vi "Main_progetto.vi"() -> ()   [LabVIEW 2019]
uses:
  <vilib>/Analysis/coordinate.llb/Angle Units.ctl
  <vilib>/Analysis/coordinate.llb/Angle Range (Degree).ctl
  <vilib>/Analysis/coordinate.llb/Wrap Angle (scalar).vi
  <vilib>/Analysis/coordinate.llb/Wrap Angle (array).vi
  <vilib>/Analysis/4window.llb/Triangle Window (DBL).vi
  <vilib>/Analysis/4window.llb/Hanning Window (DBL).vi
  <vilib>/Analysis/2dsp.llb/Real FFT.vi
  <vilib>/Analysis/4window.llb/AllCosWindow (DBL).vi
  <vilib>/Utility/file.llb/Write Delimited Spreadsheet (string).vi
  <vilib>/measure/NI_MABase.lvlib
  <vilib>/Analysis/NI_AALBase.lvlib
  <vilib>/Analysis/NI_AAL_Angle.lvlib
  <vilib>/Analysis/NI_AALPro.lvlib
panel:
  in  "IpDFT?":bool
  in  "Tw [s]":dbl=0.04
  in  "Finestra":enum16{"Rettangolare", "Triangolare", "Hann"}(ring)=enum."Hann"
  in  "Tab Control":T1(tab)=enum."Finestratura e DFT"
  in  "Gradino_FASE?":bool
  in  "Gradi innalzamento[°]":dbl=10.0
  in  "Gradino_AMP?":bool
  in  "Variazione Percentuale [%]":dbl=10.0
  in  "t0[s]":dbl=1.0
  in  "f_mp":dbl=5.0
  in  "f_ma":dbl=5.0
  in  "Ka":dbl
  in  "Kx":dbl=0.1
  out "Segnale + Fronti PPS":waveform(dbl)[](graph)=[{"t0"=timestamp(3664183274 s since 1904-01-01), "dt"=0.0001, "Y"=array[10000 elements]}, {"t0"=timestamp(3664183274 s since 1904-01-01), "dt"=0.0001, "Y"=array[10000 elements]}]
  in  "Tipo di Segnale":T2(ring)
  in  "#PPS":dbl=50.0
  in  "Tempo Osservazione [s]":dbl=1.0
  in  "fs [Campioni/s]":i32=10000
  in  "Fase iniziale [°]":dbl
  in  "Frequenza [Hz]":dbl=50.0
  in  "Ampiezza [V]":dbl=5.0
  out "#Campioni":dbl=10000.0
  out "Indici Fronte PPS":i32[](array[numeric])=[200, 400, 600, 800, 1000, 1200, 1400, 1600, 1800, 2000, 2200, 2400, 2600, 2800, 3000, 3200, 3400, 3600, 3800, 4000, 4200, 4400, 4600, 4800, 5000, 5200, 5400, 5600, 5800, 6000, 6200, 6400, 6600, 6800, 7000, 7200, 7400, 7600, 7800, 8000, 8200, 8400, 8600, 8800, 9000, 9200, 9400, 9600, 9800]
  out "Ampiezza":waveform(dbl)(graph)={"t0"=timestamp(3664183274 s since 1904-01-01), "dt"=0.0001, "Y"=array[10000 elements]}
  out "Fase":waveform(dbl)(graph)={"t0"=timestamp(3664183274 s since 1904-01-01), "dt"=0.0001, "Y"=array[10000 elements]}
  out "Frequenza":waveform(dbl)(graph)={"t0"=timestamp(3664183274 s since 1904-01-01), "dt"=0.0001, "Y"=array[10000 elements]}
  out "current time":timestamp=timestamp(3664183274 s since 1904-01-01)
  in  "Ampiezza [% Fondamentale]":dbl=10.0
  in  "Indice Fondamentale":i32=2
  in  "Armonica?":bool
  in  "Fase Arm [°]":dbl=90.0
  in  "Rumore?":bool
  in  "SNR[dB]":dbl=20.0
  out "tf":dbl
  in  "Rf":dbl=1.0
  in  "f1":dbl=45.0
  in  "f2":dbl=55.0
  in  "ti":dbl=1.0
  out "#cicli nominali in Tw":dbl=2.0
  out "FFT Modulo":dbl[](graph)=[0.2004284654332121, 0.2771875769031888, 2.4289122109023182, 0.14855120479340944, 0.06711997171608222, 0.040910071789265014, 0.02860978087861402, 0.021693180356150216, 0.01735076197275401, 0.014410410758733146, 0.012305673610300686, 0.010733350016924947, 0.00951833235799889, 0.00855331737321674, 0.007769333424100193, 0.007120260807923017, 0.0065742159898430855, 0.006108519981725259, 0.005706637938963746, 0.00535625155471345, 0.005048007477321536, 0.004774682642835479, 0.004530614276304571, 0.004311302288502253, 0.004113126580084852, 0.00393314254154195, 0.003768930776703592, 0.003618485076706068, 0.0034801278028881856, 0.003352445195024498, 0.0032342373581623067, 0.0031244791961971886, 0.0030222896028904455, 0.0029269069476381758, 0.002837669407508284, 0.0027539990648302085, 0.002675388955918328, 0.002601392451414109, 0.0025316144927998267, 0.0024657043171863423, 0.002403349383395278, 0.002344270273936035, 0.002288216394479222, 0.0022349623286919426, 0.0021843047348013493, 0.0021360596917879443, 0.002090060421054105, 0.00204615532277344, 0.0020042062772505946, 0.001964087170384628, 0.0019256826093842281, 0.0018888868006225951, 0.0018536025661511036, 0.0018197404793038816, 0.0017872181027114862, 0.001755959314936195, 0.0017258937138572004, 0.001696956086625786, 0.0016690859379216423, 0.0016422270688726094, 0.001616327200532036, 0.001591337636447327, 0.0015672129596478706, 0.0015439107600185866, 0.0015213913885452437, 0.0014996177353782815, 0.0014785550290975637, 0.0014581706547211013, 0.0014384339886332367, 0.0014193162484461821, 0.0014007903562823843, 0.0013828308142269058, 0.0013654135904523955, 0.0013485160151872353, 0.001332116685420944, 0.0013161953775471433, 0.0013007329671651806, 0.0012857113553683764, 0.001271113400898479, 0.0012569228576905357, 0.0012431243171547128, 0.0012297031550276365, 0.001216645482162153, 0.0012039380989247045, 0.0011915684531612913, 0.0011795246009920425, 0.001167795170576942, 0.001156369328410249, 0.0011452367479786612, 0.0011343875806037183, 0.001123812428279146, 0.001113502318356494, 0.0011034486799218212, 0.0010936433217333095, 0.0010840784116325608, 0.0010747464572455527, 0.001065640287970658, 0.001056753038069751, 0.0010480781308387342, 0.0010396092637684215, 0.0010313403946015805, 0.0010232657282498885, 0.0010153797044930933, 0.001007676986416554, 0.001000152449526727, 0.0009928011715113465, 0.0009856184225786999, 0.0009785996563626902, 0.000971740501352381, 0.000965036752774153, 0.0009584843649591924, 0.0009520794441221284, 0.0009458182415198593, 0.0009396971470064985, 0.0009337126829168997, 0.0009278614982866133, 0.0009221403633728558, 0.0009165461644668986, 0.0009110758989654318, 0.0009057266707131591, 0.0009004956855705209, 0.0008953802472070446, 0.0008903777531326384, 0.0008854856908649937, 0.0008807016343617123, 0.0008760232405762775, 0.0008714482462017238, 0.0008669744645753551, 0.0008625997827203524, 0.0008583221585377279, 0.0008541396181274819, 0.0008500502532454137, 0.0008460522188465611, 0.0008421437308167747, 0.0008383230637082276, 0.0008345885486464955, 0.0008309385713546284, 0.0008273715701607699, 0.0008238860342263808, 0.0008204805017666113, 0.0008171535583750218, 0.0008139038354303445, 0.0008107300085636059, 0.0008076307962000254, 0.0008046049581566672, 0.0008016512943030512, 0.0007987686433104722, 0.0007959558813671575, 0.0007932119210777466, 0.0007905357103051015, 0.0007879262310841407, 0.0007853824986460356, 0.0007829035603848542, 0.0007804884949445779, 0.000778136411309154, 0.0007758464479433901, 0.0007736177719647078, 0.0007714495783565443, 0.0007693410891995958, 0.0007672915529728252, 0.0007653002438213416, 0.0007633664609190352, 0.0007614895278423043, 0.0007596687919177555, 0.0007579036236858507, 0.0007561934163169723, 0.0007545375850835884, 0.0007529355668558493, 0.0007513868196077115, 0.0007498908219539457, 0.0007484470727029584, 0.0007470550904400135, 0.0007457144131051204, 0.0007444245976283224, 0.0007431852195461328, 0.0007419958726416369, 0.0007408561686510532, 0.0007397657368926213, 0.0007387242240051496, 0.0007377312936482901, 0.0007367866262287676, 0.0007358899186506904, 0.0007350408840707933, 0.0007342392516738983, 0.0007334847664536476, 0.0007327771890147256, 0.0007321162953945121, 0.0007315018768564688, 0.0007309337397749528, 0.0007304117054513229, 0.0007299356099701171, 0.0007295053041087158, 0.000729120653183006, 0.0007287815369684133, 0.0007284878495977631, 0.000728239499483278, 0.0007280364092437072, 0.0007278785156508138, 0.0007277657695728192, 0.0007276981359433338, 0.0007276755937394297, 0.0007276981359433338, 0.0007277657695728192, 0.0007278785156508138, 0.0007280364092437072, 0.000728239499483278, 0.0007284878495977631, 0.0007287815369684133, 0.000729120653183006, 0.0007295053041087158, 0.0007299356099701171, 0.0007304117054513229, 0.0007309337397749528, 0.0007315018768564688, 0.0007321162953945121, 0.0007327771890147256, 0.0007334847664536476, 0.0007342392516738983, 0.0007350408840707933, 0.0007358899186506904, 0.0007367866262287676, 0.0007377312936482901, 0.0007387242240051496, 0.0007397657368926213, 0.0007408561686510532, 0.0007419958726416369, 0.0007431852195461328, 0.0007444245976283224, 0.0007457144131051204, 0.0007470550904400135, 0.0007484470727029584, 0.0007498908219539457, 0.0007513868196077115, 0.0007529355668558493, 0.0007545375850835884, 0.0007561934163169723, 0.0007579036236858507, 0.0007596687919177555, 0.0007614895278423043, 0.0007633664609190352, 0.0007653002438213416, 0.0007672915529728252, 0.0007693410891995958, 0.0007714495783565443, 0.0007736177719647078, 0.0007758464479433901, 0.000778136411309154, 0.0007804884949445779, 0.0007829035603848542, 0.0007853824986460356, 0.0007879262310841407, 0.0007905357103051015, 0.0007932119210777466, 0.0007959558813671575, 0.0007987686433104722, 0.0008016512943030512, 0.0008046049581566672, 0.0008076307962000254, 0.0008107300085636059, 0.0008139038354303445, 0.0008171535583750218, 0.0008204805017666113, 0.0008238860342263808, 0.0008273715701607699, 0.0008309385713546284, 0.0008345885486464955, 0.0008383230637082276, 0.0008421437308167747, 0.0008460522188465611, 0.0008500502532454137, 0.0008541396181274819, 0.0008583221585377279, 0.0008625997827203524, 0.0008669744645753551, 0.0008714482462017238, 0.0008760232405762775, 0.0008807016343617123, 0.0008854856908649937, 0.0008903777531326384, 0.0008953802472070446, 0.0009004956855705209, 0.0009057266707131591, 0.0009110758989654318, 0.0009165461644668986, 0.0009221403633728558, 0.0009278614982866133, 0.0009337126829168997, 0.0009396971470064985, 0.0009458182415198593, 0.0009520794441221284, 0.0009584843649591924, 0.000965036752774153, 0.000971740501352381, 0.0009785996563626902, 0.0009856184225786999, 0.0009928011715113465, 0.001000152449526727, 0.001007676986416554, 0.0010153797044930933, 0.0010232657282498885, 0.0010313403946015805, 0.0010396092637684215, 0.0010480781308387342, 0.001056753038069751, 0.001065640287970658, 0.0010747464572455527, 0.0010840784116325608, 0.0010936433217333095, 0.0011034486799218212, 0.001113502318356494, 0.001123812428279146, 0.0011343875806037183, 0.0011452367479786612, 0.001156369328410249, 0.001167795170576942, 0.0011795246009920425, 0.0011915684531612913, 0.0012039380989247045, 0.001216645482162153, 0.0012297031550276365, 0.0012431243171547128, 0.0012569228576905357, 0.001271113400898479, 0.0012857113553683764, 0.0013007329671651806, 0.0013161953775471433, 0.001332116685420944, 0.0013485160151872353, 0.0013654135904523955, 0.0013828308142269058, 0.0014007903562823843, 0.0014193162484461821, 0.0014384339886332367, 0.0014581706547211013, 0.0014785550290975637, 0.0014996177353782815, 0.0015213913885452437, 0.0015439107600185866, 0.0015672129596478706, 0.001591337636447327, 0.001616327200532036, 0.0016422270688726094, 0.0016690859379216423, 0.001696956086625786, 0.0017258937138572004, 0.001755959314936195, 0.0017872181027114862, 0.0018197404793038816, 0.0018536025661511036, 0.0018888868006225951, 0.0019256826093842281, 0.001964087170384628, 0.0020042062772505946, 0.00204615532277344, 0.002090060421054105, 0.0021360596917879443, 0.0021843047348013493, 0.0022349623286919426, 0.002288216394479222, 0.002344270273936035, 0.002403349383395278, 0.0024657043171863423, 0.0025316144927998267, 0.002601392451414109, 0.002675388955918328, 0.0027539990648302085, 0.002837669407508284, 0.0029269069476381758, 0.0030222896028904455, 0.0031244791961971886, 0.0032342373581623067, 0.003352445195024498, 0.0034801278028881856, 0.003618485076706068, 0.003768930776703592, 0.00393314254154195, 0.004113126580084852, 0.004311302288502253, 0.004530614276304571, 0.004774682642835479, 0.005048007477321536, 0.00535625155471345, 0.005706637938963746, 0.006108519981725259, 0.0065742159898430855, 0.007120260807923017, 0.007769333424100193, 0.00855331737321674, 0.00951833235799889, 0.010733350016924947, 0.012305673610300686, 0.014410410758733146, 0.01735076197275401, 0.021693180356150216, 0.02860978087861402, 0.040910071789265014, 0.06711997171608222, 0.14855120479340944, 2.4289122109023182, 0.2771875769031888]
  in  "Freq Nom [Hz]":dbl=50.0
  out "Finestre":dbl[][](graph)
  out "Nw":i32=400
  out "Errore Ampiezza":waveform(dbl)(graph)={"t0"=timestamp(3664183274 s since 1904-01-01), "dt"=0.02, "Y"=[-2.783764844462926, -2.0643275081794954, -1.0948068040687353, -0.1185268667778594, 0.6260382249297258, 0.9612665795103048, 0.8083537049149925, 0.2031572038769447, -0.7109376274646095, -1.7128090786989603, -2.553584527277426, -3.018941014895642, -2.9880383189683712, -2.468950838768471, -1.5962499435632438, -0.5917665408033912, 0.2957958814533157, 0.8523582805366736, 0.9463029139744528, 0.5556087136146104, -0.22777463298394807, -1.2165051574097774, -2.1682944281056216, -2.8435115639072883, -3.0682120621809794, -2.783764844462926, -2.0643275081794776, -1.0948068040687708, -0.11852686677787716, 0.6260382249297258, 0.9612665795103226, 0.8083537049149925, 0.2031572038769447, -0.7109376274645918, -1.7128090786989425, -2.553584527277444, -3.018941014895624, -2.9880383189683712, -2.468950838768471, -1.5962499435632616, -0.591766540803409, 0.2957958814533157, 0.8523582805366381, 0.9463029139744883, 0.5556087136146282, -0.22777463298389478, -1.2165051574097419, -2.1682944281056926, -2.8435115639072706]}
  out "Errore Fase":waveform(dbl)(graph)={"t0"=timestamp(3664183274 s since 1904-01-01), "dt"=0.02, "Y"=[-0.9924999827672032, -1.7110408606274774, -1.9782950781677577, -1.7401357120577998, -1.0674646300828705, -0.12793342028531995, 0.8562237454428079, 1.6540002345176053, 2.0717014022732627, 1.9972557434297045, 1.4354923368755657, 0.5196901501313356, -0.5154977010656481, -1.3996886023500466, -1.907559062866504, -1.9206641317435214, -1.4494430035050243, -0.6179136942558117, 0.37334049987567397, 1.291927161654316, 1.9197643004517762, 2.098729550599465, 1.771865154751795, 1.0089419265595867, 1.0132179603049215e-13, -0.9924999827664926, -1.711040860628188, -1.9782950781673136, -1.7401357120615302, -1.0674646300826929, -0.12793342028372123, 0.8562237454401211, 1.6540002345162952, 2.071701402273396, 1.997255743427706, 1.4354923368743222, 0.5196901501328899, -0.5154977010668915, -1.399688602349869, -1.9075590628678363, -1.9206641317449424, -1.4494430035063566, -0.6179136942584762, 0.3733404998801815, 1.2919271616545158, 1.919764300447624, 2.0987295505939474, 1.7718651547519726, 1.00894192655972]}
  out "TVE (Total vector error)":waveform(dbl)(graph)={"t0"=timestamp(3664183274 s since 1904-01-01), "dt"=0.02, "Y"=[2.9507581085918675, 2.6699442744155264, 2.2515062053425523, 1.7431166101168498, 1.2403738519873968, 0.9698235534221632, 1.180032412638305, 1.6680782166788377, 2.183280452227935, 2.618070021606387, 2.9204070891337692, 3.0620138182269923, 3.0308695047565517, 2.8295662779157382, 2.475601509722746, 2.0042942995676443, 1.481403950898688, 1.054317408745175, 1.0179347508680092, 1.4096194593664053, 1.9310278865612676, 2.4147065727130195, 2.7879836372364273, 3.0124022833472104, 3.0682120621809794, 2.9507581085916126, 2.669944274415972, 2.2515062053421486, 1.7431166101206395, 1.2403738519872842, 0.9698235534219634, 1.180032412636331, 1.6680782166775265, 2.1832804522280598, 2.6180700216048662, 2.9204070891332026, 3.062013818227213, 3.0308695047567613, 2.829566277915625, 2.4756015097237265, 2.0042942995689703, 1.4814039509000156, 1.0543174087467533, 1.0179347508697123, 1.409619459366593, 1.93102788655714, 2.414706572708266, 2.7879836372365867, 3.0124022833472384]}
  out "Errore Frequenza":waveform(dbl)(graph)={"t0"=timestamp(3664183274.02 s since 1904-01-01), "dt"=0.02, "Y"=[-57.17966626252036, -21.267414891852354, 18.952120180031784, 53.529463885624295, 74.76551811420507, 78.3167388524788, 63.485035859386585, 33.239602791795164, -5.924197298384115, -44.70371150065944, -72.8772224572296, -82.37763177344704, -70.36167628813672, -40.415047120767156, -1.0428682455412286, 37.498585924147676, 66.17099994641507, 78.8815024283096, 73.09880394018364, 49.96169204815715, 14.241602101130013, -26.011042159602482, -60.71150148331128, -80.28904745239629, -78.98063913800968, -57.17966626252036, -21.267414891852354, 18.952120180031784, 53.529463885624295, 74.76551811420507, 78.3167388524788, 63.485035859386585, 33.23960279180227, -5.924197298384115, -44.70371150065944, -72.8772224572296, -82.37763177343993, -70.36167628813672, -40.41504712077426, -1.0428682455412286, 37.49858592415478, 66.17099994642217, 78.88150242831671, 73.09880394018364, 49.96169204815004, 14.241602101130013, -26.011042159595377, -60.71150148331128]}
  out "Ampiezza Misurata":waveform(dbl)[](graph)=[{"t0"=timestamp(3664183274 s since 1904-01-01), "dt"=0.02, "Y"=[4.860811757776854, 4.896783624591025, 4.945259659796563, 4.994073656661107, 5.031301911246486, 5.048063328975515, 5.04041768524575, 5.010157860193847, 4.9644531186267695, 4.914359546065052, 4.872320773636129, 4.849052949255218, 4.850598084051581, 4.8765524580615764, 4.920187502821838, 4.97041167295983, 5.014789794072666, 5.042617914026834, 5.047315145698723, 5.0277804356807305, 4.988611268350803, 4.939174742129511, 4.891585278594719, 4.857824421804636, 4.846589396890951, 4.860811757776854, 4.896783624591026, 4.9452596597965615, 4.994073656661106, 5.031301911246486, 5.048063328975516, 5.04041768524575, 5.010157860193847, 4.96445311862677, 4.914359546065053, 4.872320773636128, 4.849052949255219, 4.850598084051581, 4.8765524580615764, 4.920187502821837, 4.9704116729598296, 5.014789794072666, 5.042617914026832, 5.047315145698724, 5.027780435680731, 4.988611268350805, 4.939174742129513, 4.891585278594715, 4.8578244218046365]}, {"t0"=timestamp(3664183274 s since 1904-01-01), "dt"=0.02, "Y"=[5.0, 5.0, 5.0, 5.0, 5.0, 5.0, 5.0, 5.0, 5.0, 5.0, 5.0, 5.0, 5.0, 5.0, 5.0, 5.0, 5.0, 5.0, 5.0, 5.0, 5.0, 5.0, 5.0, 5.0, 5.0, 5.0, 5.0, 5.0, 5.0, 5.0, 5.0, 5.0, 5.0, 5.0, 5.0, 5.0, 5.0, 5.0, 5.0, 5.0, 5.0, 5.0, 5.0, 5.0, 5.0, 5.0, 5.0, 5.0, 5.0]}]
  out "Fase Misurata":waveform(dbl)[](graph)=[{"t0"=timestamp(3664183274 s since 1904-01-01), "dt"=0.02, "Y"=[-0.2612524121148551, -0.5197652331806407, -0.7737651876432275, -1.0227110062693092, -1.2673117077367457, -1.5092438079259523, -1.7507296485558532, -1.9940792959522873, -2.2412296965619127, -2.4933015654375374, -2.750246611790268, -3.010732045944878, 3.0107739704355416, 2.7506046491355156, 2.494198532243169, 2.2427400692672315, 1.9961248682624204, 1.7531127490677307, 1.5116978787218631, 1.2695563330524675, 1.02450729215326, 0.7749695323675265, 0.5203734761219104, 0.2614168315527921, 1.0132179603049215e-15, -0.2612524121148537, -0.519765233180639, -0.7737651876432263, -1.022711006269308, -1.2673117077367444, -1.5092438079259507, -1.7507296485558517, -1.9940792959522862, -2.2412296965619114, -2.493301565437536, -2.750246611790266, -3.0107320459448768, 3.0107739704355434, 2.750604649135518, 2.4941985322431703, 2.242740069267232, 1.996124868262421, 1.753112749067732, 1.5116978787218656, 1.2695563330524695, 1.0245072921532612, 0.7749695323675282, 0.5203734761219122, 0.26141683155279344]}, {"t0"=timestamp(3664183274 s since 1904-01-01), "dt"=0.02, "Y"=[-0.2513274122871829, -0.5026548245743658, -0.7539822368615496, -1.0053096491487317, -1.2566370614359172, -1.5079644737230993, -1.7592918860102813, -2.0106192982974633, -2.2619467105846454, -2.5132741228718345, -2.7646015351590236, -3.0159289474461914, 3.0159289474461985, 2.7646015351590165, 2.5132741228718345, 2.2619467105846667, 2.0106192982974704, 1.7592918860102884, 1.5079644737231064, 1.2566370614359244, 1.0053096491487423, 0.7539822368615319, 0.5026548245743925, 0.25132741228719624, 0.0, -0.25132741228718913, -0.502654824574357, -0.7539822368615532, -1.0053096491486926, -1.2566370614359172, -1.5079644737231135, -1.7592918860102529, -2.010619298297449, -2.2619467105846454, -2.513274122871813, -2.7646015351590094, -3.0159289474462057, 3.0159289474462128, 2.7646015351590165, 2.5132741228718487, 2.261946710584681, 2.0106192982974846, 1.7592918860103168, 1.5079644737230637, 1.2566370614359244, 1.005309649148785, 0.7539822368615887, 0.5026548245743925, 0.25132741228719624]}]
  out "Frequenza Misurata":waveform(dbl)[](graph)=[{"t0"=timestamp(3664183274.02 s since 1904-01-01), "dt"=0.02, "Y"=[47.94282033373748, 47.97873258510815, 48.01895212018003, 48.053529463885624, 48.074765518114205, 48.07831673885248, 48.06348503585939, 48.033239602791795, 47.994075802701616, 47.95529628849934, 47.92712277754277, 47.91762236822655, 47.92963832371186, 47.95958495287923, 47.99895713175446, 48.03749858592415, 48.066170999946415, 48.07888150242831, 48.073098803940184, 48.04996169204816, 48.01424160210113, 47.9739889578404, 47.93928849851669, 47.919710952547604, 47.92101936086199, 47.94282033373748, 47.97873258510815, 48.01895212018003, 48.053529463885624, 48.074765518114205, 48.07831673885248, 48.06348503585939, 48.0332396027918, 47.994075802701616, 47.95529628849934, 47.92712277754277, 47.91762236822656, 47.92963832371186, 47.959584952879226, 47.99895713175446, 48.037498585924155, 48.06617099994642, 48.07888150242832, 48.073098803940184, 48.04996169204815, 48.01424160210113, 47.973988957840405, 47.93928849851669]}, {"t0"=timestamp(3664183274.02 s since 1904-01-01), "dt"=0.02, "Y"=[48.0, 48.0, 48.0, 48.0, 48.0, 48.0, 48.0, 48.0, 48.0, 48.0, 48.0, 48.0, 48.0, 48.0, 48.0, 48.0, 48.0, 48.0, 48.0, 48.0, 48.0, 48.0, 48.0, 48.0, 48.0, 48.0, 48.0, 48.0, 48.0, 48.0, 48.0, 48.0, 48.0, 48.0, 48.0, 48.0, 48.0, 48.0, 48.0, 48.0, 48.0, 48.0, 48.0, 48.0, 48.0, 48.0, 48.0, 48.0]}]
  out "Errore max Ampiezza[%]":dbl=0.9612665795103226
  out "Errore max TVE[%]":dbl=3.0682120621809794
  out "Errore max Fase[crad]":dbl=2.098729550599465
  out "Errore Medio Fase[crad]":dbl=0.06411413578686515
  out "Errore max Frequenza [mHz]":dbl=78.88150242831671
  out "Errore Medio Frequenza [mHz]":dbl=3.318118470634346
  out "Errore Medio Ampiezza[%]":dbl=-0.9977148663108252
  out "Errore Medio TVE[%]":dbl=2.1404587015174017
  out "Array String":string[][](array[string])
  in  "format string M3":string="%8.4f"
  in  "format string M2":string="%8.5f"
  in  "format string M1":string="%6.3f"
  out "error out":errorcluster
  in  "Header":string[][](array[string])=[["Timestamp", "Ampiezza", "Fase", "Frequenza"], ["", "[V]", "[rad]", "[Hz]"]]
  in  "Nome File":string="file"
  in  "Save?":bool
  # "PER USARE L'IpDFT \nABILITARE LA FINESTRA DI HANN!"
  # "Parametri Segnale"
  # "Parametri Modulazione"
  # "Disturbi"
  # "Gradino"
  # "Rampa di Frequenza"
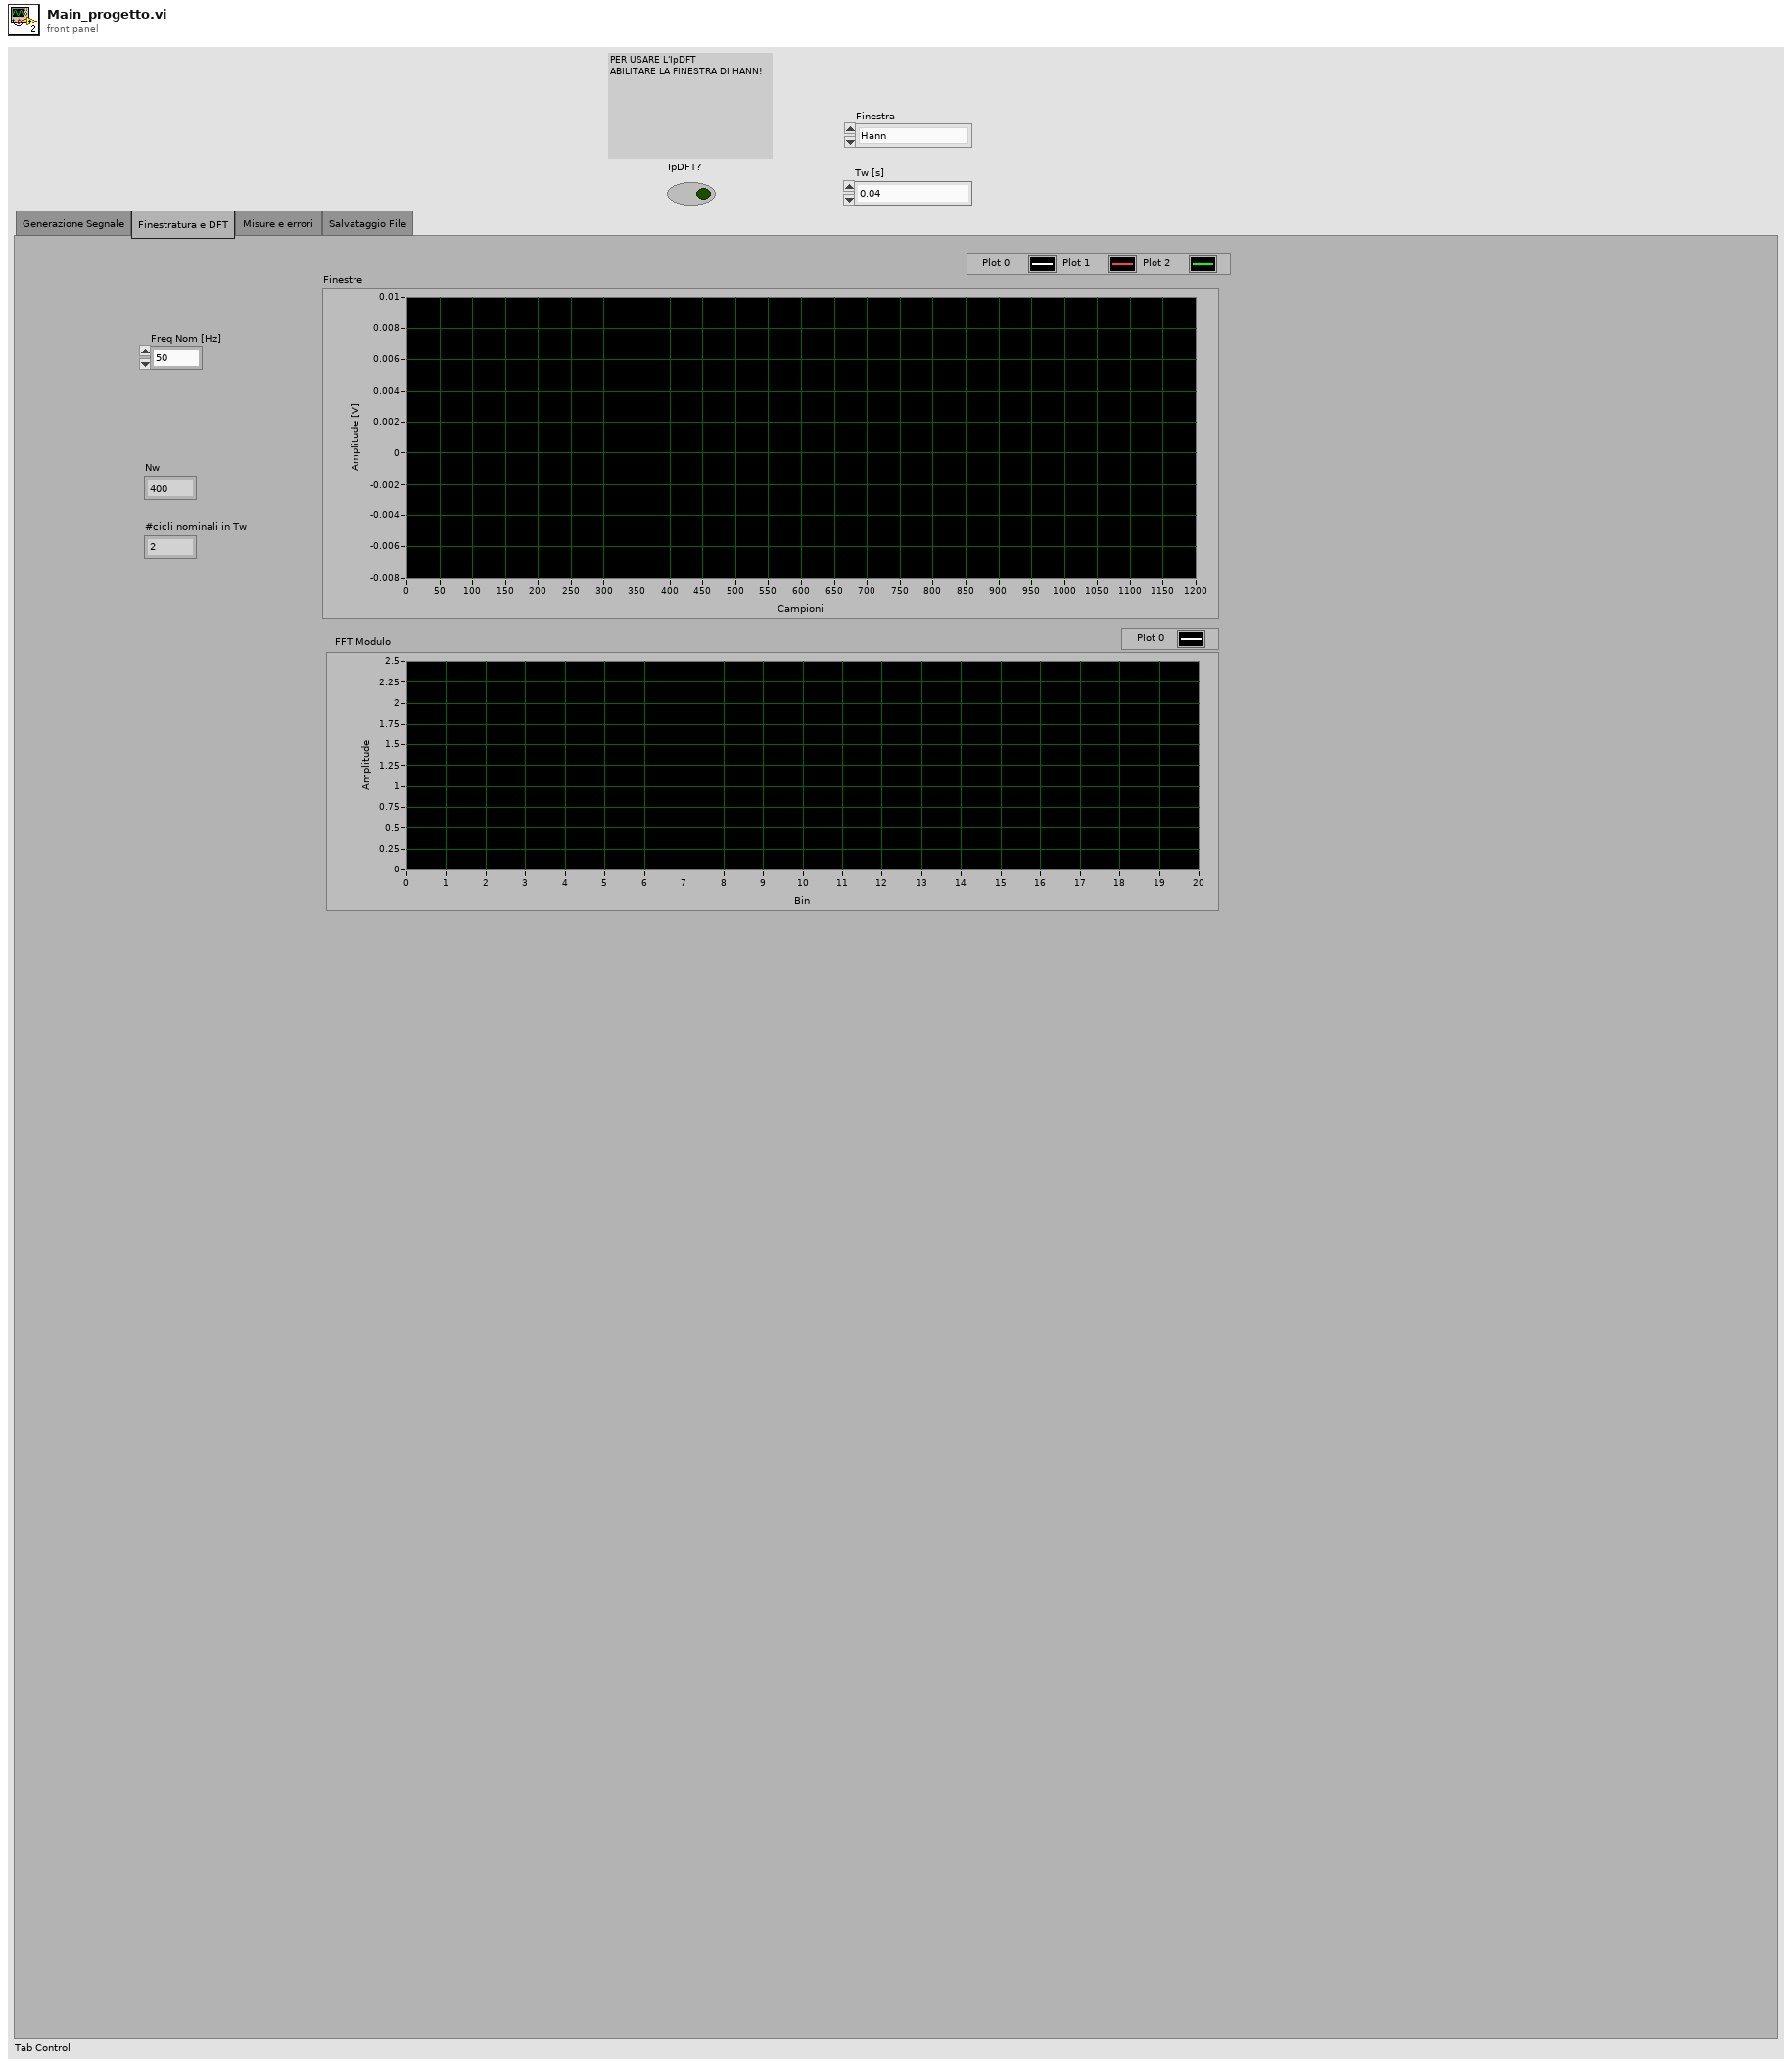
[diagram p1: front panel]
types:
  T1 = enum32{"Generazione Segnale", "Finestratura e DFT", "Misure e errori ", "Salvataggio File"}
  T2 = enum16{"Stazionario", "Modulazione", "Rampa di frequenza"}
  T3 = typedef "NI_AAL_Angle.lvlib/Angle Range (Degree).ctl" = u16
  T4 = typedef "NI_AAL_Angle.lvlib/Angle Units.ctl" = i32
  T5 = typedef "LVDateTimeRec.ctl" = cluster{"fractional second":dbl, "second":i32, "minute":i32, "hour":i32, "day of month":i32, "month":i32, "year":i32, "day of week":i32, "day of year":i32, "DST":i32}
  T6 = cluster{waveform(dbl), waveform(dbl), waveform(dbl)}
  T7 = cluster{waveform(ext), waveform(ext), waveform(dbl), i32[]}
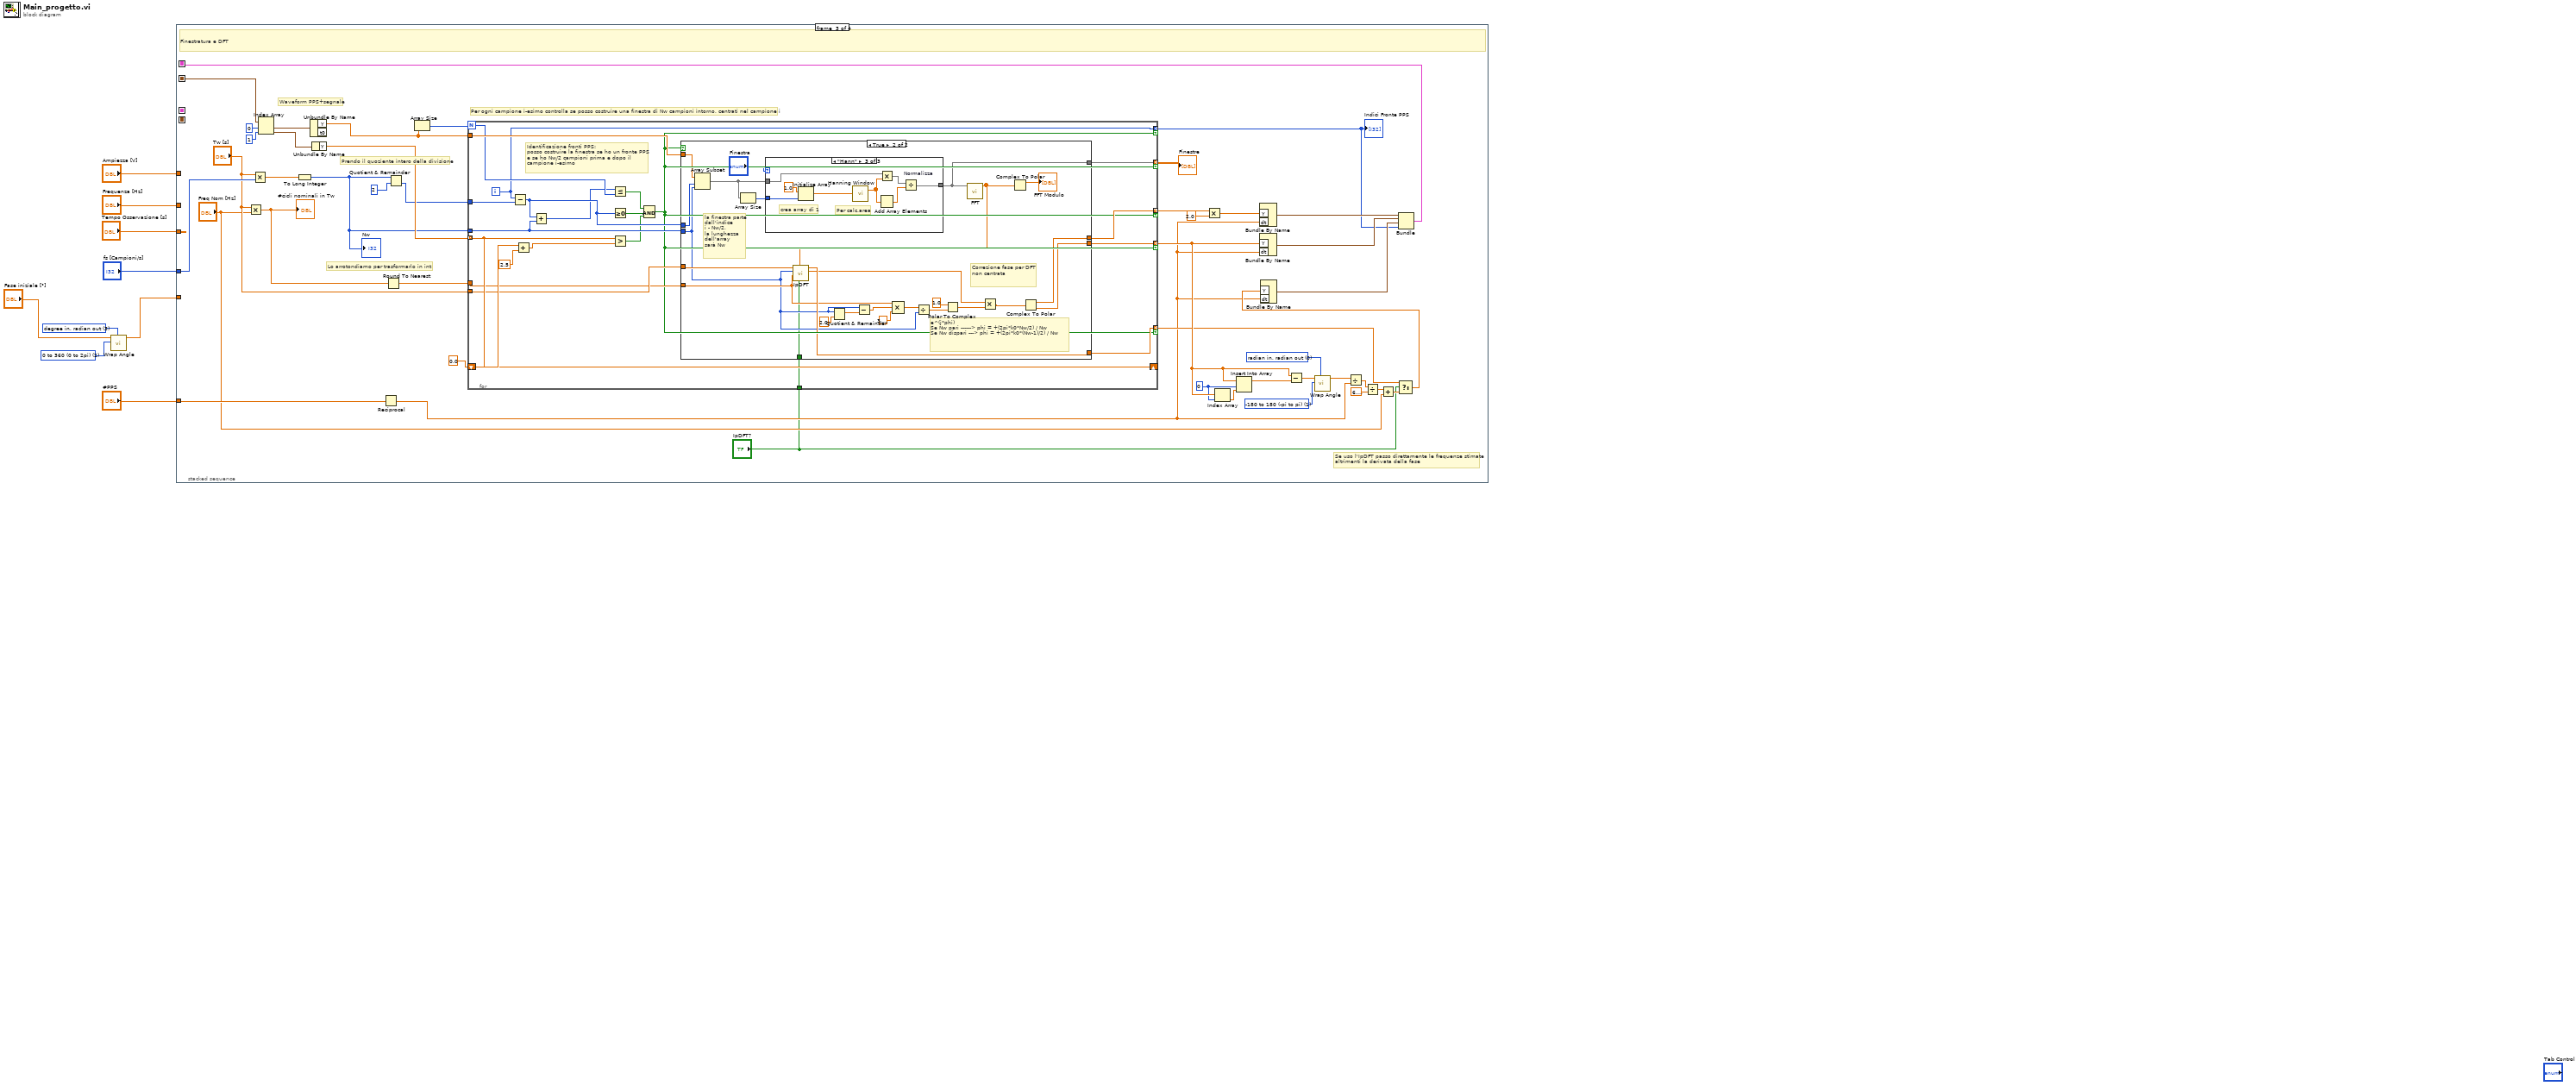
[diagram p0: block diagram]
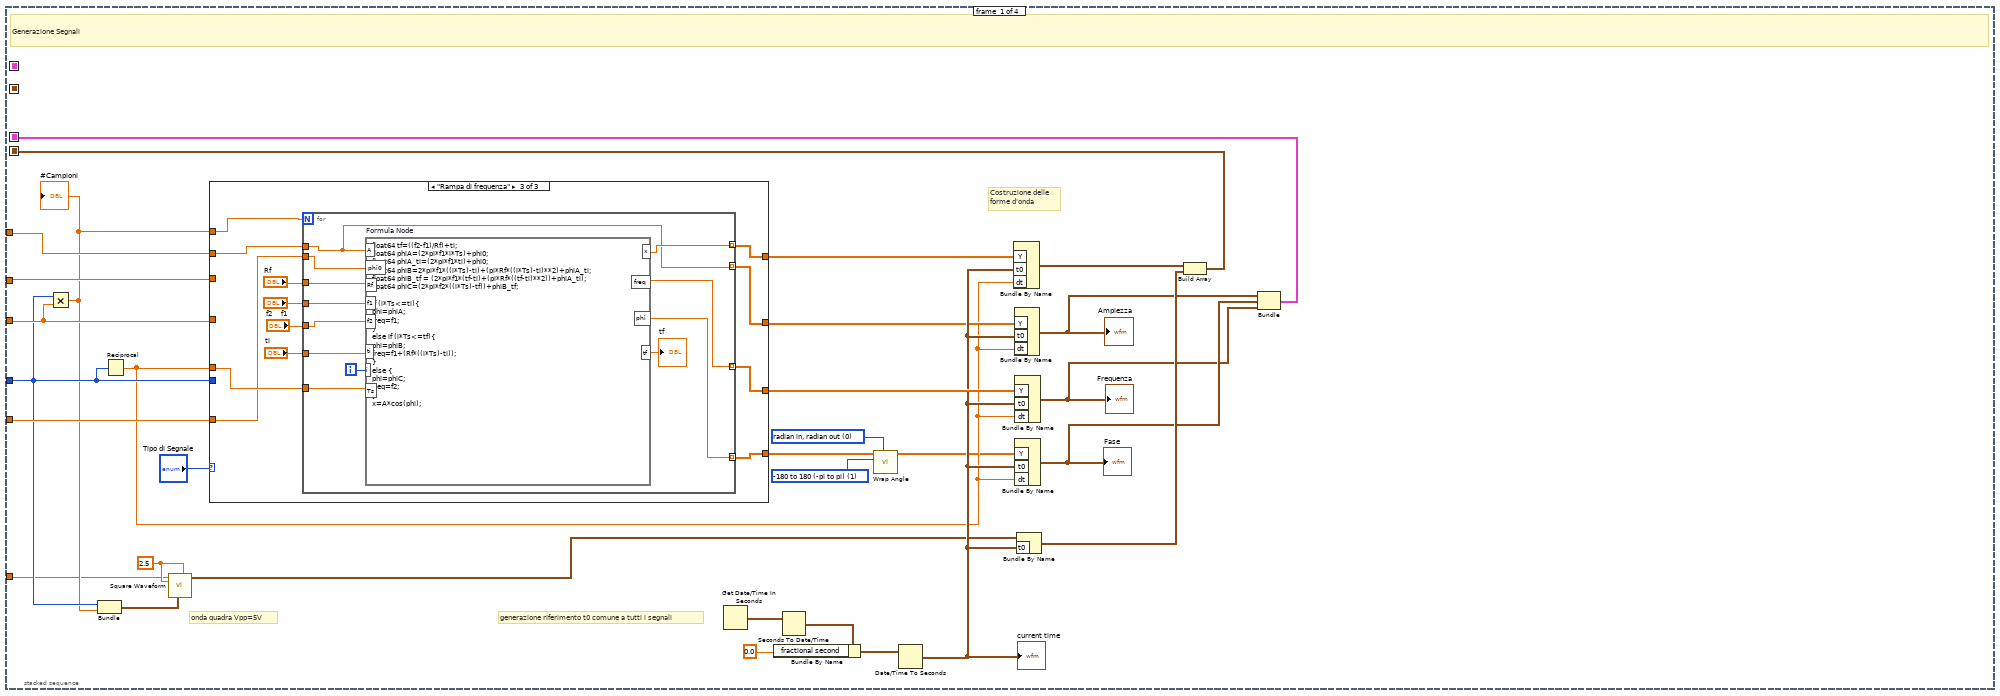
[diagram p2: hidden frame]
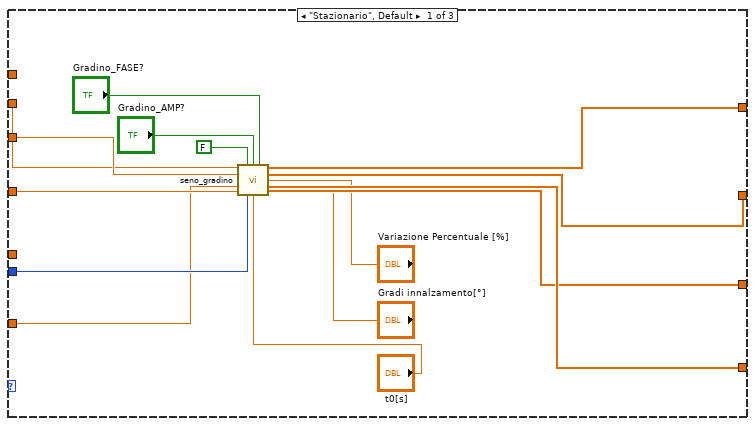
[diagram p3: hidden frame]
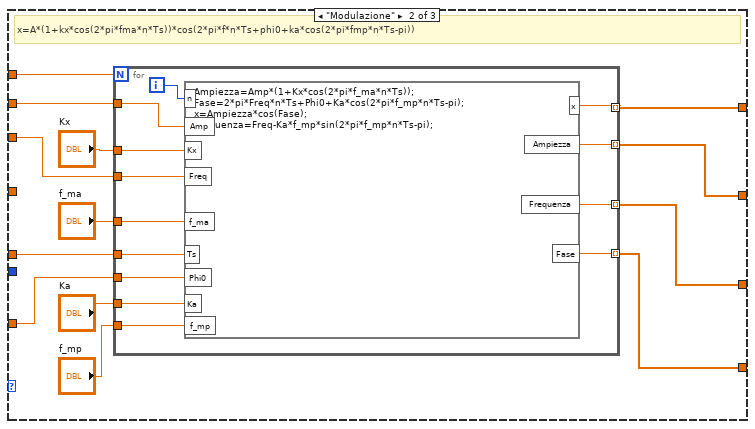
[diagram p4: hidden frame]
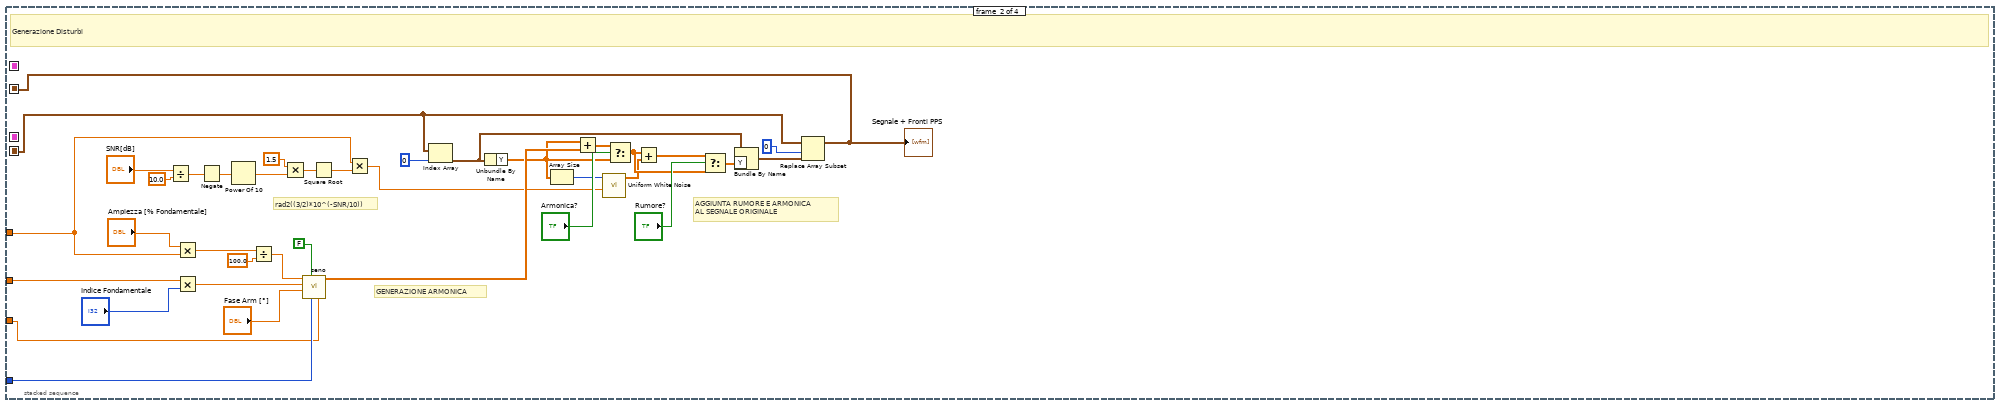
[diagram p5: hidden frame]
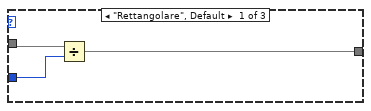
[diagram p7: hidden frame]
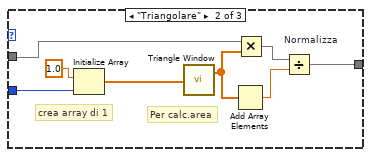
[diagram p8: hidden frame]
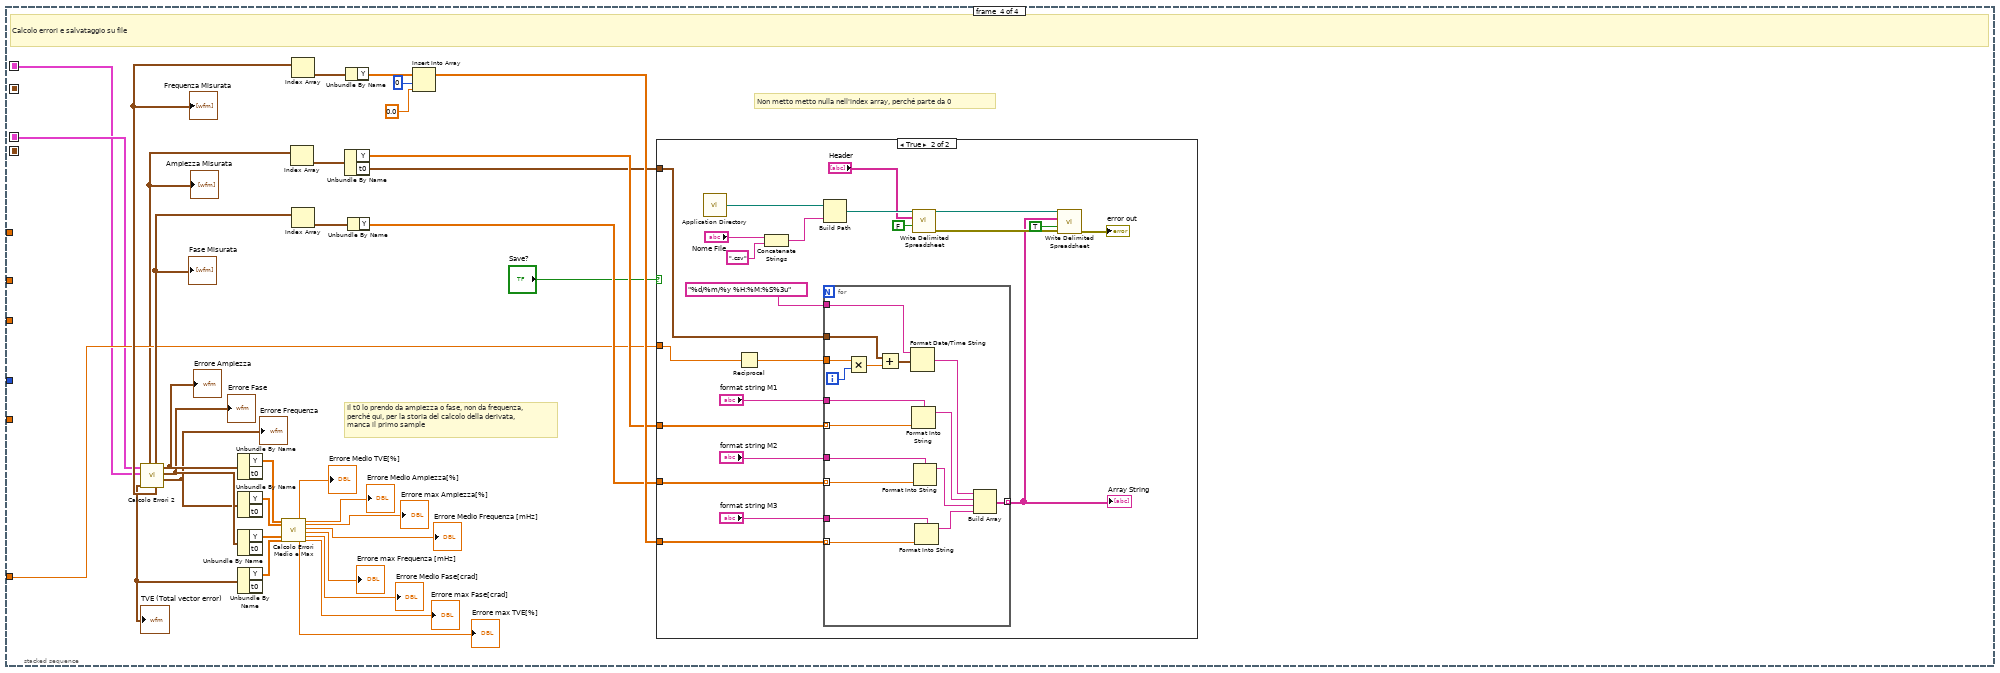
[diagram p9: hidden frame]
diagram:
  w3 = T3 2 items=["none", "-180 to 180 (-pi to pi)", "0 to 360 (0 to 2pi)"] ("angle range")
  w4 = T4 3 items=["radian in, radian out", "radian in, degree out", "degree in, degree out", "degree in, radian out"] ("angle units")
  n1 = call-poly <vilib>:"Wrap Angle.vi"("angle units"=w4, "angle range"=w3, "angle in"="Fase iniziale [°]") -> ("angle out"=w1:dbl)  [unwired: 7 in, 1 out]
  n2 = stacked-sequence {
    seq-local: [w28 _ _ _] -> [_ w110 _ _]
    seq-local: [_ w107 _ _] -> [_ _ w186 _]
    seq-local: [w14 _ _ _] -> [_ _ _ w255]
    seq-local: [_ _ w152 _] -> [_ _ _ w254]
    tunnel: "fs [Campioni/s]" -> [w31 w140 w177 _]
    tunnel: "Tempo Osservazione [s]" -> [w32 w139 _ _]
    tunnel: "Ampiezza [V]" -> [w35 w106 _ _]
    tunnel: "Frequenza [Hz]" -> [w34 w134 _ _]
    tunnel: w1 -> [w33 _ _ _]
    tunnel: "#PPS" -> [w18 _ w159 w275]
    frame #0 {
      w24 = T4 0 items=["radian in, radian out", "radian in, degree out", "degree in, degree out", "degree in, radian out"] ("angle units")
      w25 = T3 1 items=["none", "-180 to 180 (-pi to pi)", "0 to 360 (0 to 2pi)"] ("angle range")
      w40 = 2.5 ("amplitude")
      # "Costruzione delle\nforme d'onda"
      # "onda quadra Vpp=5V"
      # "generazione riferimento t0 comune a tutti i segnali"
      # "Generazione Segnali"
      n3 = Multiply(x=w31, y=w32) -> (x*y=w21:dbl)
      "#Campioni" <- w21
      n4 = Bundle("fs [Campioni/s]"=w31, w21) -> (w39:cluster{"fs [Campioni/s]":i32, dbl})  [unwired: 1 in]
      n5 = Reciprocal(x=w31) -> (1/x=w19:dbl)
      n6 = call <vilib>:"Square Waveform.vi"("offset"=w40, "sampling info"=w39, "amplitude"=w40, "frequency"=w18) -> ("signal out"=w10:waveform(dbl))  [unwired: 6 in, 1 out]
      n7 = case shown="\"Rampa di frequenza\"" "Tipo di Segnale" {
        tunnel: w35 -> [w49 w63 w87]
        tunnel: w34 -> [w50 w62 _]
        tunnel: w33 -> [w47 w61 w86]
        tunnel: w32 -> [w52 _ _]
        tunnel: w31 -> [w51 _ _]
        tunnel: w21 -> [_ w68 w89]
        tunnel: w19 -> [_ w60 w88]
        tunnel: [w48 w59 w83] -> w20
        tunnel: [w54 w58 w84] -> w26
        tunnel: [w53 w57 w85] -> w27
        tunnel: [w41 w56 w82] -> w15
        frame "Stazionario", Default {
          n8 = call "seno_gradino.vi"("ampiezza [V]"=w49, "scelta_funzione"=FALSE, "Gradino_AMP?"="Gradino_AMP?", "Gradino_FASE?"="Gradino_FASE?", "frequenza[Hz]"=w50, "Variazione Percentuale [%]"="Variazione Percentuale [%]", "fase[°]"=w47, "Gradi innalzamento[°]"="Gradi innalzamento[°]", "rate [sample/s]"=w51, "t0[s]"="t0[s]", "lunghezza finestra[s]"=w52) -> ("Waveform Graph"=w41:dbl[], "Ampiezza"=w48:dbl[], "Fase"=w54:dbl[], "Frequenza"=w53:dbl[])  [unwired: 1 in]
        }
        frame "Modulazione" {
          # "x=A*(1+kx*cos(2*pi*fma*n*Ts))*cos(2*pi*f*n*Ts+phi0+ka*cos(2*pi*fmp*n*Ts-pi))"
          n9 = for {
            N: w68 -> [_]
            tunnel: "Kx" -> [w81]
            tunnel: "Ka" -> [w80]
            tunnel: "f_ma" -> [w79]
            tunnel: "f_mp" -> [w78]
            tunnel: w63 -> [w77]
            tunnel: w62 -> [w76]
            tunnel: w61 -> [w75]
            tunnel: w60 -> [w73]
            tunnel: [w72] -> w56 mode=indexing
            tunnel: [w71] -> w59 mode=indexing
            tunnel: [w69] -> w58 mode=indexing
            tunnel: [w70] -> w57 mode=indexing
            i -> [w74]
            n10 = formula code="Ampiezza=Amp*(1+Kx*cos(2*pi*f_ma*n*Ts));\nFase=2*pi*Freq*n*Ts+Phi0+Ka*cos(2*pi*f_mp*n*Ts-pi);\nx=Ampiezza*cos(Fase);\nFrequenza=Freq-Ka*f_mp*sin(2*pi*f_mp*n*Ts-pi);"("Amp"=w77, "Kx"=w81, "f_ma"=w79, "n"=w74, "Ts"=w73, "Freq"=w76, "Phi0"=w75, "Ka"=w80, "f_mp"=w78) -> ("x"=w72:dbl, "Ampiezza"=w71:dbl, "Fase"=w69:dbl, "Frequenza"=w70:dbl)
          }
        }
        frame "Rampa di frequenza" {
          n11 = for {
            N: w89 -> [_]
            tunnel: [w105] -> w82 mode=indexing
            tunnel: [w103] -> w84 mode=indexing
            tunnel: [w104] -> w85 mode=indexing
            tunnel: "Rf" -> [w100]
            tunnel: "f1" -> [w99]
            tunnel: "f2" -> [w98]
            tunnel: "ti" -> [w97]
            tunnel: w88 -> [w96]
            tunnel: w87 -> [w94]
            tunnel: w86 -> [w95]
            tunnel: [w94] -> w83 mode=indexing
            i -> [w101]
            n12 = formula code="float64 tf=((f2-f1)/Rf)+ti;\nfloat64 phiA=(2*pi*f1*i*Ts)+phi0;\nfloat64 phiA_ti=(2*pi*f1*ti)+phi0;\nfloat64 phiB=2*pi*f1*((i*Ts)-ti)+(pi*Rf*((i*Ts)-ti)**2)+phiA_ti;\nfloat64 phiB_tf = (2*pi*f1*(tf-ti)+(pi*Rf*((tf-ti)**2))+phiA_ti);\nfloat64 phiC=(2*pi*f2*((i*Ts)-tf))+phiB_tf;\n\nif (i*Ts<=ti){ \nphi=phiA;\nfreq=f1;\n}\nelse if (i*Ts<=tf){ \nphi=phiB;\nfreq=f1+(Rf*((i*Ts)-ti));\n}\nelse {\nphi=phiC;\nfreq=f2;\n}\nx=A*cos(phi);"("A"=w94, "phi0"=w95, "Rf"=w100, "f1"=w99, "f2"=w98, "ti"=w97, "i"=w101, "Ts"=w96) -> ("freq"=w104:dbl, "phi"=w103:dbl, "x"=w105:dbl, "tf"=→"tf":dbl)
          }
        }
      }
      n13 = Get Date/Time In Seconds() -> (seconds since 1Jan1904=w38:timestamp)
      n14 = Seconds To Date/Time(time stamp (now)=w38) -> (date time rec=w37:T5)  [unwired: 1 in]
      n15 = Bundle By Name(cluster=w37, "fractional second"=0.0) -> (w23:T5)
      n16 = call-poly <vilib>:"Wrap Angle.vi"("angle units"=w24, "angle range"=w25, "Angle In"=w26) -> ("Angle Out"=w16:dbl[])  [unwired: 7 in, 1 out]
      n17 = Date/Time To Seconds(2:w23) -> (0:w22:timestamp)  [unwired: 1 in]
      "current time" <- w22
      n18 = Bundle By Name("Y"=w15, "t0"=w22, "dt"=w19) -> (w30:waveform(dbl))  [unwired: 1 in]
      n19 = Bundle By Name("Y"=w20, "t0"=w22, "dt"=w19) -> (w13:waveform(dbl))  [unwired: 1 in]
      "Ampiezza" <- w13
      n20 = Bundle By Name("Y"=w27, "t0"=w22, "dt"=w19) -> (w11:waveform(dbl))  [unwired: 1 in]
      "Frequenza" <- w11
      n21 = Bundle By Name("Y"=w16, "t0"=w22, "dt"=w19) -> (w12:waveform(dbl))  [unwired: 1 in]
      "Fase" <- w12
      n22 = Bundle By Name(cluster=w10, "t0"=w22) -> (w29:waveform(dbl))
      n23 = Build Array(w30, w29) -> (w28:waveform(dbl)[])
      n24 = Bundle(w13, w12, w11) -> (w14:T6)  [unwired: 1 in]
    }
    frame #1 {
      # "AGGIUNTA RUMORE E ARMONICA \nAL SEGNALE ORIGINALE"
      # "GENERAZIONE ARMONICA"
      # "rad2((3/2)*10^(-SNR/10))"
      # "Generazione Disturbi"
      n25 = Divide(x="SNR[dB]", y=10.0) -> (x/y=w125:dbl)
      n26 = Multiply(x="Ampiezza [% Fondamentale]", y=w106) -> (x*y=w138:dbl)
      n27 = Multiply(x=w134, y="Indice Fondamentale") -> (x*y=w132:dbl)
      n28 = Negate(x=w125) -> (-x=w124:dbl)
      n29 = Power Of 10(x=w124) -> (10^x=w123:dbl)
      n30 = Divide(x=w138, y=100.0) -> (x/y=w136:dbl)
      n31 = Multiply(x=1.5, y=w123) -> (x*y=w121:dbl)
      n32 = call "seno.vi"("lunghezza finestra[s]"=w139, "rate [sample/s]"=w140, "scelta_funzione"=FALSE, "fase[°]"="Fase Arm [°]", "frequenza[Hz]"=w132, "ampiezza [V]"=w136) -> ("Waveform Graph"=w130:dbl[])  [unwired: 2 in, 3 out]
      n33 = Square Root(x=w121) -> (sqrt(x)=w120:dbl)
      n34 = Multiply(x=w106, y=w120) -> (x*y=w119:dbl)
      n35 = Index Array "Index Array"(array=w110, index=0) -> (element=w112:waveform(dbl))
      n36 = Unbundle By Name ("Get Waveform Components")(w112) -> ("Y"=w118:dbl[])
      n37 = Array Size(array=w118) -> (size(s)=w117:i32)
      n38 = Add(x=w118, y=w130) -> (x+y=w128:dbl[])
      n39 = call <vilib>:"Uniform White Noise.vi"("amplitude"=w119, "samples"=w117) -> ("uniform white noise"=w114:dbl[])  [unwired: 8 in, 1 out]
      n40 = Select(t=w128, s="Armonica?", f=w118) -> (s? t:f=w115:dbl[])
      n41 = Add(x=w115, y=w114) -> (x+y=w113:dbl[])
      n42 = Select(t=w113, s="Rumore?", f=w115) -> (s? t:f=w111:dbl[])
      n43 = Bundle By Name(cluster=w112, "Y"=w111) -> (w108:waveform(dbl))
      n44 = Replace Array Subset(array=w110, new element=w108, index=0) -> (w107:waveform(dbl)[])
      "Segnale + Fronti PPS" <- w107
    }
    frame #2 {
      w158 = 0 ("index")
      w164 = T4 0 items=["radian in, radian out", "radian in, degree out", "degree in, degree out", "degree in, radian out"] ("angle units")
      w165 = T3 1 items=["none", "-180 to 180 (-pi to pi)", "0 to 360 (0 to 2pi)"] ("angle range")
      # "Lo arrotondiamo per trasformarlo in int"
      # "Se uso l'IpDFT passo direttamente le frequenze stimate\naltrimenti la derivata della fase"
      # "Per ogni campione i-esimo controlla se posso costruire una finestra di Nw campioni intorno, centrati nel campione i"
      # "Waveform PPS+segnale"
      # "Prendo il quoziente intero della divisione"
      # "Finestratura e DFT"
      n45 = Multiply(x="Tw [s]", y="Freq Nom [Hz]") -> (x*y=w145:dbl)
      "#cicli nominali in Tw" <- w145
      n46 = Multiply(x="Tw [s]", y=w177) -> (x*y=w157:dbl)
      n47 = Index Array "Index Array"(array=w186, index #1=0 ("index"), index #2=1 ("index")) -> (element #1=w183:waveform(dbl), element #2=w182:waveform(dbl))
      n48 = To Long Integer(number=w157) -> (32bit integer=w144:i32)
      "Nw" <- w144
      n49 = Unbundle By Name(w183) -> ("Y"=w180:dbl[])  [unwired: 1 out]
      n50 = Unbundle By Name(w182) -> ("Y"=w179:dbl[])
      n51 = Reciprocal(x=w159) -> (1/x=w148:dbl)
      n52 = Round To Nearest(number=w145) -> (nearest integer value=w146:dbl)
      n53 = Quotient & Remainder(x=w144, y=2) -> (floor(x/y)=w175:i32)  [unwired: 1 out]
      n54 = Array Size(array=w180) -> (size(s)=w181:i32)
      n55 = for {
        N: w181 -> [w200]
        tunnel: w180 -> [w204]
        tunnel: w179 -> [w205] mode=indexing
        shift-right: [w205] -> _
        shift-left: 0.0 -> [w208]
        tunnel: [w192] -> w160 mode=indexing if=w188
        tunnel: w144 -> [w201]
        tunnel: w175 -> [w193]
        tunnel: [w203] -> w150 mode=indexing if=w188
        tunnel: [w198] -> w147 mode=indexing if=w188
        tunnel: [w197] -> w172 mode=indexing if=w188
        tunnel: "Tw [s]" -> [w196]
        tunnel: w146 -> [w195]
        tunnel: [w194] -> w151 mode=indexing if=w188
        tunnel: "IpDFT?" -> [w187]
        i -> [w192]
        # "Identificazione fronti PPS:\nposso costruire la finestra se ho un fronte PPS\ne se ho Nw/2 campioni prima e dopo il\ncampione i-esimo"
        n56 = Subtract(x=w192, y=w193) -> (x-y=w202:i32)
        n57 = Add(x=w208, y=2.5) -> (x+y=w206:dbl)
        n58 = Add(x=w202, y=w201) -> (x+y=w199:i32)
        n59 = Less Or Equal?(x=w199, y=w200) -> (x <= y?=w191:bool)
        n60 = Greater Or Equal To 0?(x=w202) -> (x >= 0?=w190:bool)
        n61 = Greater?(x=w205, y=w206) -> (0:w189:bool)
        n62 = Compound Arithmetic op=AND(w191, w190, w189) -> (w188:bool)
        n63 = case shown="True" w188 {
          tunnel: w204 -> [_ w230]
          tunnel: w201 -> [_ w210]
          tunnel: w202 -> [_ w233]
          tunnel: [_ w228] -> w203
          tunnel: [_ w226] -> w198
          tunnel: [_ w225] -> w197
          tunnel: w196 -> [_ w224]
          tunnel: w195 -> [_ w213]
          tunnel: [_ w222] -> w194
          tunnel: w187 -> [_ w209]
          frame False {
          }
          frame True {
            # "Correzione fase per DFT \nnon centrata"
            # "e^(j*phi)\nSe Nw pari ------> phi = +(2pi*k0*Nw/2) / Nw\nSe Nw dispari ---> phi = +(2pi*k0*(Nw-1)/2) / Nw"
            # "la finestra parte\ndall'indice\ni - Nw/2,\nla lunghezza\ndell'array \nsarà Nw"
            n64 = Array Subset(array=w230, index=w233, length=w210) -> (w229:dbl[])
            n65 = Array Size(array=w229) -> (size(s)=w231:i32)
            n66 = case shown="\"Hann\"" "Finestra" {
              tunnel: w231 -> [w236 w239 w252]
              tunnel: [w235 w241 w247] -> w228
              tunnel: w229 -> [w234 w240 w250]
              frame "Rettangolare", Default {
                n67 = Divide(x=w234, y=w236) -> (x/y=w235:dbl[])
              }
              frame "Triangolare" {
                # "crea array di 1"
                # "Per calc.area"
                n68 = Initialize Array(1.0 ("element"), w239) -> (w238:dbl[])
                n69 = call-poly <vilib>:"Triangle Window.vi"("X"=w238) -> ("Windowed X"=w237:dbl[])  [unwired: 1 out]
                n70 = Add Array Elements(numeric array=w237) -> (sum=w242:dbl)
                n71 = Multiply(x=w240, y=w237) -> (x*y=w243:dbl[])
                n72 = Divide "Normalizza"(x=w243, y=w242) -> (x/y=w241:dbl[])
              }
              frame "Hann" {
                # "crea array di 1"
                # "Per calc.area"
                n73 = Initialize Array(1.0 ("element"), w252) -> (w245:dbl[])
                n74 = call-poly <vilib>:"Hanning Window.vi"("X"=w245) -> ("Windowed X"=w246:dbl[])  [unwired: 1 out]
                n75 = Add Array Elements(numeric array=w246) -> (sum=w248:dbl)
                n76 = Multiply(x=w250, y=w246) -> (x*y=w249:dbl[])
                n77 = Divide "Normalizza"(x=w249, y=w248) -> (x/y=w247:dbl[])
              }
            }
            n78 = Quotient & Remainder(x=w210, y=2.0) -> (x-y*floor(x/y)=w212:dbl)  [unwired: 1 out]
            n79 = Subtract(x=w210, y=w212) -> (x-y=w218:dbl)
            n80 = Compound Arithmetic op=MULTIPLY(w213, w218, 3.141592653589793) -> (w217:dbl)
            n81 = Divide(x=w217, y=w210) -> (x/y=w216:dbl)
            n82 = Polar To Complex(1:w216, 2:1.0 ("r")) -> (0:w220:cdb)
            n83 = call-poly <vilib>:"FFT.vi"("X"=w228) -> ("FFT {X}"=w223:cdb[])  [unwired: 9 in, 1 out]
            n84 = call "IpDFT.vi"("IpDFT?"=w209, "FFT{X}"=w223, "k0"=w213, "Nw"=w210, "Tw"=w224) -> ("X_stimata[f0]"=w215:cxt, "f0 stimato"=w222:dbl)  [unwired: 5 in]
            n85 = Multiply(x=w215, y=w220) -> (x*y=w214:cxt)
            n86 = Complex To Polar(r * e^(i*theta)=w223) -> (r=→"FFT Modulo":dbl[])  [unwired: 1 out]
            n87 = Complex To Polar(r * e^(i*theta)=w214) -> (r=w226:ext, theta=w225:ext)
          }
        }
      }
      "Indici Fronte PPS" <- w160
      "Finestre" <- w150
      n88 = Multiply(x=w147, y=2.0) -> (x*y=w174:ext[])
      n89 = Index Array(array=w172, index=w158) -> (element=w173:ext)
      n90 = Insert Into Array "Insert Into Array"(array=w172, index=w158, new element=w173) -> (w171:ext[])
      n91 = Bundle By Name("Y"=w174, "dt"=w148) -> (w163:waveform(ext))  [unwired: 1 in]
      n92 = Bundle By Name("Y"=w172, "dt"=w148) -> (w162:waveform(ext))  [unwired: 1 in]
      n93 = Subtract(x=w172, y=w171) -> (x-y=w167:ext[])
      n94 = call-poly <vilib>:"Wrap Angle.vi"("angle units"=w164, "angle range"=w165, "Angle In"=w167) -> ("Angle Out"=w166:dbl[])  [unwired: 7 in, 1 out]
      n95 = Divide(x=w166, y=w148) -> (x/y=w170:dbl[])
      n96 = Divide(x=w170, y=6.283185307179586) -> (x/y=w168:dbl[])
      n97 = Add(x=w168, y="Freq Nom [Hz]") -> (x+y=w155:dbl[])
      n98 = Select(t=w151, s="IpDFT?", f=w155) -> (s? t:f=w149:dbl[])
      n99 = Bundle By Name("Y"=w149, "dt"=w148) -> (w161:waveform(dbl))  [unwired: 1 in]
      n100 = Bundle(w163, w162, w161, w160) -> (w152:T7)  [unwired: 1 in]
    }
    frame #3 {
      # "Il t0 lo prendo da ampiezza o fase, non da frequenza,\nperché qui, per la storia del calcolo della derivata,\nmanca il primo sample"
      # "Non metto metto nulla nell'index array, perché parte da 0"
      # "Calcolo errori e salvataggio su file"
      n101 = call "Calcolo Errori 2.vi"("Misure"=w254, "Riferimenti"=w255) -> ("TVE"=w271:waveform(dbl), "Errore Frequenza"=w272:waveform(dbl), "Errore Fase"=w273:waveform(dbl), "Errore Ampiezza"=w274:waveform(dbl), "Frequenza Misurata"=w277:waveform(dbl)[], "Fase Misurata"=w276:waveform(dbl)[], "Ampiezza Misurata"=w258:waveform(dbl)[])  [unwired: 3 in]
      "Errore Ampiezza" <- w274
      "Errore Fase" <- w273
      "Errore Frequenza" <- w272
      "TVE (Total vector error)" <- w271
      "Ampiezza Misurata" <- w258
      "Fase Misurata" <- w276
      "Frequenza Misurata" <- w277
      n102 = Unbundle By Name(w274) -> ("Y"=w270:dbl[])  [unwired: 1 out]
      n103 = Unbundle By Name(w272) -> ("Y"=w269:dbl[])  [unwired: 1 out]
      n104 = Unbundle By Name(w273) -> ("Y"=w268:dbl[])  [unwired: 1 out]
      n105 = Unbundle By Name(w271) -> ("Y"=w267:dbl[])  [unwired: 1 out]
      n106 = call "Calcolo Errori Medio e Max.vi"("Misure Errore Ampiezza[%]"=w270, "Misure Errore Frequenza[mHz]"=w269, "Misure Errore Fase[crad]"=w268, "Misure Errore TVE[%]"=w267) -> ("Errore Medio TVE[%]"=→"Errore Medio TVE[%]":dbl, "Errore max TVE[%]"=→"Errore max TVE[%]":dbl, "Errore Medio Ampiezza[%]"=→"Errore Medio Ampiezza[%]":dbl, "Errore max Ampiezza[%]"=→"Errore max Ampiezza[%]":dbl, "Errore Medio Frequenza [mHz]"=→"Errore Medio Frequenza [mHz]":dbl, "Errore max Frequenza [mHz]"=→"Errore max Frequenza [mHz]":dbl, "Errore Medio Fase[crad]"=→"Errore Medio Fase[crad]":dbl, "Errore max Fase[crad]"=→"Errore max Fase[crad]":dbl)  [unwired: 8 in]
      n107 = Index Array(array=w258) -> (element=w257:waveform(dbl))  [unwired: 1 in]
      n108 = Index Array(array=w277) -> (element=w284:waveform(dbl))  [unwired: 1 in]
      n109 = Index Array(array=w276) -> (element=w285:waveform(dbl))  [unwired: 1 in]
      n110 = Unbundle By Name(w257) -> ("Y"=w279:dbl[], "t0"=w278:timestamp)
      n111 = Unbundle By Name(w284) -> ("Y"=w283:dbl[])
      n112 = Unbundle By Name(w285) -> ("Y"=w280:dbl[])
      n113 = Insert Into Array(array=w283, index=0, new element=0.0 ("new element/subarray")) -> (w281:dbl[])
      n114 = case shown="True" "Save?" {
        tunnel: w281 -> [_ w290]
        tunnel: w280 -> [_ w286]
        tunnel: w279 -> [_ w288]
        tunnel: w278 -> [_ w289]
        tunnel: w275 -> [_ w287]
        frame False {
        }
        frame True {
          n115 = call <vilib>:"Application Directory.vi"() -> ("Application Directory"=w307:path)
          n116 = Reciprocal(x=w287) -> (1/x=w293:dbl)
          n117 = Concatenate Strings("Nome File", ".csv" ("string")) -> (w304:string)
          n118 = Build Path(base path=w307, name or relative path=w304) -> (appended path=w303:path)
          n119 = for {
            tunnel: w288 -> [w324] mode=indexing
            tunnel: w286 -> [w323] mode=indexing
            tunnel: w290 -> [w308] mode=indexing
            tunnel: "format string M1" -> [w322]
            tunnel: "format string M2" -> [w309]
            tunnel: "format string M3" -> [w321]
            tunnel: [w317] -> w291 mode=indexing
            tunnel: w293 -> [w315]
            tunnel: w289 -> [w313]
            tunnel: "%d/%m/%y %H:%M:%S%3u" ("time format string (%c)") -> [w312]
            i -> [w316]
            n120 = Multiply(x=w315, y=w316) -> (x*y=w314:dbl)
            n121 = Add(x=w313, y=w314) -> (x+y=w311:timestamp)
            n122 = Format Date/Time String(time format string (%c)=w312, seconds (now)=w311) -> (date/time string=w310:string)  [unwired: 1 in]
            n123 = Format Into String(format string=w322, w324) -> (resulting string=w320:string)  [unwired: 2 in, 1 out]
            n124 = Format Into String(format string=w309, w323) -> (resulting string=w319:string)  [unwired: 2 in, 1 out]
            n125 = Format Into String(format string=w321, w308) -> (resulting string=w318:string)  [unwired: 2 in, 1 out]
            n126 = Build Array(w310, w320, w319, w318) -> (w317:string[])
          }
          "Array String" <- w291
          n127 = call-poly <vilib>:"Write Delimited Spreadsheet.vi"("file path (dialog if empty)"=w303, "2D data"="Header", "append to file? (new file:F)"=FALSE) -> ("new file path (Not A Path if cancelled)"=w300:path, "error out"=w299:errorcluster)  [unwired: 11 in]
          n128 = call-poly <vilib>:"Write Delimited Spreadsheet.vi"("file path (dialog if empty)"=w300, "2D data"=w291, "append to file? (new file:F)"=TRUE, "error in (no error)"=w299) -> ("error out"=→"error out":errorcluster)  [unwired: 10 in, 1 out]
        }
      }
    }
  }
